vi "Encoders Reset.vi"(8 "error in (no error)":errorcluster, 11 "Encoders":cluster{"Right Encoder":T1}) -> (0 "error out":errorcluster, 3 "Encoders out":cluster{"EncoderDevRef":T1})   [LabVIEW 2013]
uses:
  <vilib>/Rock Robotics/WPI/Encoder/WPI_EncoderDevRef.ctl
  <vilib>/Rock Robotics/SystemInterfaces/Encoder/FPGA_EncoderIdx.ctl
  <vilib>/Rock Robotics/SystemInterfaces/Counter/FPGA_CounterCtrSystemIndex.ctl
  <vilib>/Rock Robotics/WPI/Encoder/WPI_EncoderType.ctl
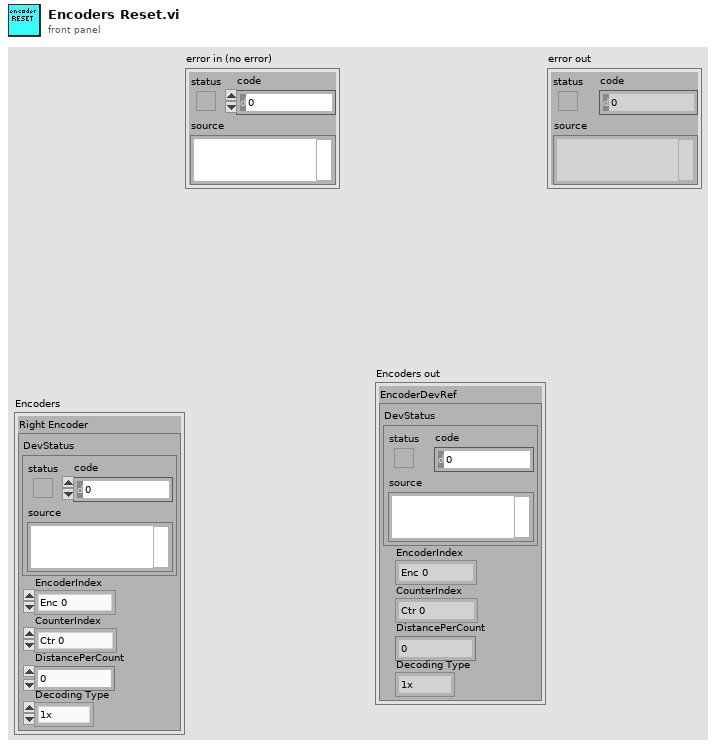
[diagram p1: front panel]
types:
  T1 = typedef "WPI_EncoderDevRef.ctl" = cluster{"DevStatus":errorcluster, "EncoderIndex":T2, "CounterIndex":T3, "DistancePerCount":dbl, "Decoding Type":T4}
  T2 = typedef "FPGA_EncoderIdx.ctl" = enum8{"Enc 0", "Enc 1", "Enc 2", "Enc 3", "Invalid"}
  T3 = typedef "FPGA_CounterCtrSystemIndex.ctl" = enum8{"Ctr 0", "Ctr 1", "Ctr 2", "Ctr 3", "Ctr 4", "Ctr 5", "Ctr 6", "Ctr 7", "Invalid"}
  T4 = typedef "WPI_EncoderType.ctl" = enum16{"1x", "2x", "4x"}
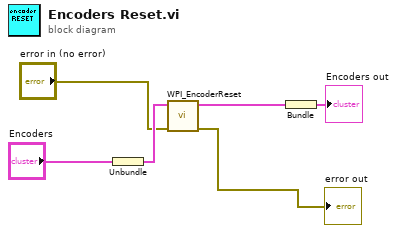
[diagram p0: block diagram]
diagram:
  n1 = Unbundle("Encoders") -> ("Right Encoder"=w5:T1)
  n2 = call <vilib>:"WPI_EncoderReset.vi"("error in (no error)"="error in (no error)", "EncoderDevRef"=w5) -> ("error out"=→"error out":errorcluster, "EncoderDevRef"=w6:T1)  [unwired: 8 in]
  n3 = Bundle("EncoderDevRef"=w6) -> (→"Encoders out":cluster{"EncoderDevRef":T1})  [unwired: 1 in]
